vi "Execute.vi"(8 "error in (no error)":errorcluster, 10 "System In":refnum<class "abs_System.lvclass">, 11 "Node in":refnum<class "Test Double Float.lvclass">) -> (0 "error out":errorcluster, 1 "Status":T1, 2 "System Out":refnum<class "abs_System.lvclass">, 3 "Node out":refnum<class "Test Double Float.lvclass">)   [LabVIEW 2021, in "BT.lvlib" / "Test Double Float.lvclass"]
uses:
  Test Double Float.lvclass
  C:/Users/Tim/Documents/LabVIEW/2021/Behaviour Tree/Source/abs_Type Leaf/abs_Type Leaf.lvclass
  abs_Node/Status.ctl
  abs_System/abs_System.lvclass
  LV_Abstract/Source/Abs_Types/Double Float/Abs_Double Float.lvclass
  C:/Users/Tim/Documents/GitHub/LV_Abstract/Source/Abs_Types/Type/Abs_Type.lvclass
  abs_Type Leaf/abs_Type Leaf.lvclass/abs_Type Leaf.ctl
  Test Double Float.lvclass/Test Double Float.ctl
  abs_Type Leaf/Properties/Read Value Class.vi
  Properties/Read Lower Limit.vi
  Properties/Read Upper Limit.vi
  Properties/Read Limit Test Type.vi
  abs_Type Leaf/Properties/Write Value Class.vi
  LV_Abstract/Source/Abs_Types/Type/Abs_Type.lvclass
  abs_Type Leaf/abs_Type Leaf.lvclass
  abs_Node/abs_Node.lvclass
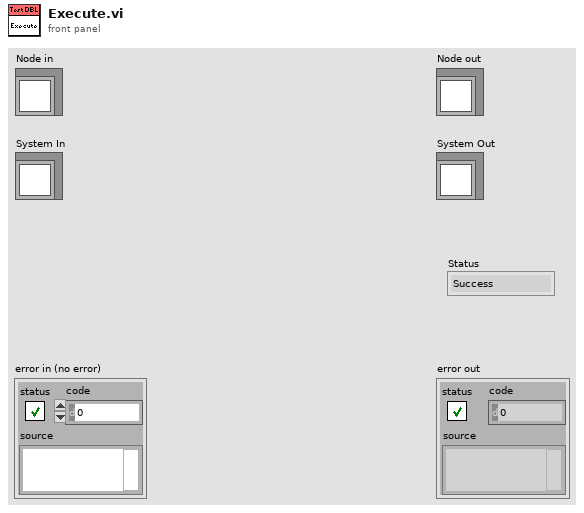
[diagram p1: front panel]
types:
  T1 = typedef "BT.lvlib/abs_Node.lvclass/Status.ctl" = enum16{"Success", "Failure", "Running"}
  T2 = typedef "BT.lvlib/Limit Test Type.ctl" = enum16{"x == Lo", "x != Lo", "x > Lo", "x < Lo", "x >= Lo", "x <= Lo", "Lo > x < Hi", "Lo >= x <= Hi", "Lo >= x < Hi", "Lo > x <= Hi", "Lo < x > Hi", "Lo <= x >= Hi", "Lo <= x > Hi", "Lo < x >= Hi", "x == Lo +/- Hi"}
  T3 = typedef "Abs_Double Float.lvclass/Type.ctl" = dbl
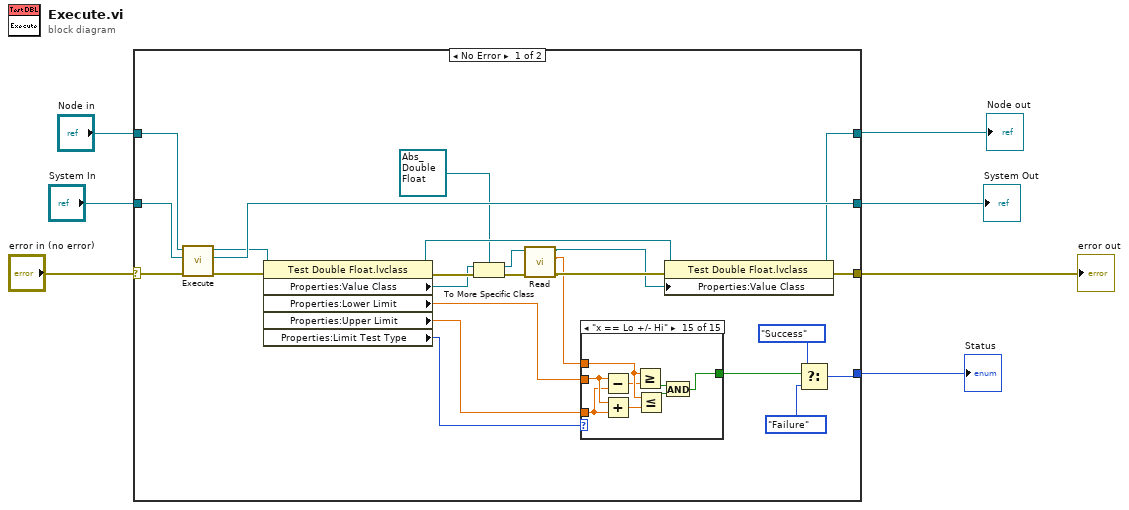
[diagram p0: block diagram]
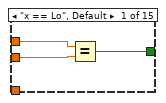
[diagram p2: hidden frame]
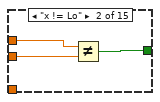
[diagram p3: hidden frame]
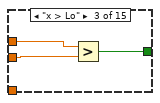
[diagram p4: hidden frame]
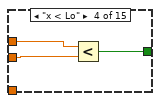
[diagram p5: hidden frame]
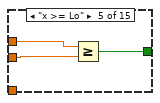
[diagram p6: hidden frame]
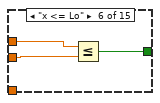
[diagram p7: hidden frame]
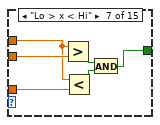
[diagram p8: hidden frame]
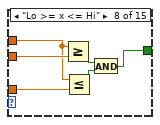
[diagram p9: hidden frame]
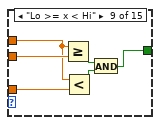
[diagram p10: hidden frame]
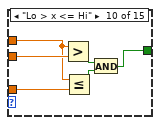
[diagram p11: hidden frame]
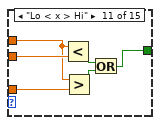
[diagram p12: hidden frame]
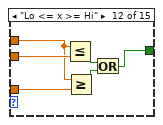
[diagram p13: hidden frame]
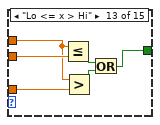
[diagram p14: hidden frame]
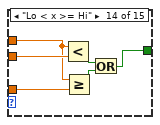
[diagram p15: hidden frame]
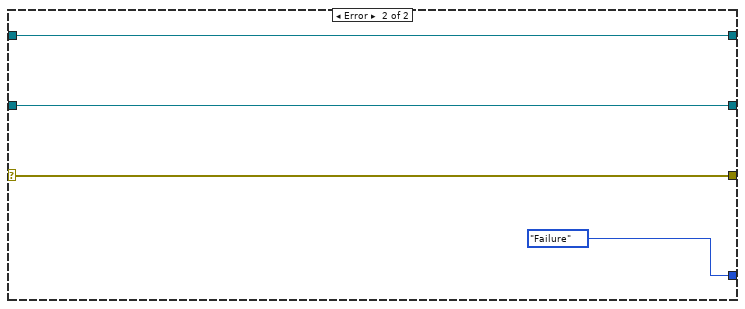
[diagram p16: hidden frame]
diagram:
  n1 = case shown="No Error" "error in (no error)" {
    selector: "error in (no error)" -> [w30 w107]
    tunnel: [w31 w108] -> w2
    tunnel: "System In" -> [w29 w108]
    tunnel: "Node in" -> [w28 w109]
    tunnel: [w24 w107] -> w4
    tunnel: [w23 w109] -> w1
    tunnel: [w20 Status."Failure" ("Status")] -> w3
    frame No Error {
      n2 = call-parent "Execute.vi"("error in (no error)"=w30, "System In"=w29, "Node in"=w28) -> ("error out"=w27:errorcluster, "System Out"=w31:refnum<class "abs_System.lvclass">, "Node out"=w26:refnum<class "Test Double Float.lvclass">)  [unwired: 5 in, 1 out]
      n3 = property class="Test Double Float.lvclass"(reference=w26, error in=w27) -> (reference out=w25:refnum<class "Test Double Float.lvclass">, error out=w11:errorcluster, "Properties:Value Class"=w10:refnum<class "Abs_Type.lvclass">, "Properties:Lower Limit"=w19:dbl, "Properties:Upper Limit"=w16:dbl, "Properties:Limit Test Type"=w17:T2)
      n4 = To More Specific Class(target class=refnum<class "Abs_Double Float.lvclass"> refnum ("Double Float.lvclass_340760 in"), reference=w10, error in=w11) -> (specific class reference=w8:refnum<class "Abs_Double Float.lvclass">, error out=w12:errorcluster)
      n5 = call-dynamic "Read.vi"("error in (no error)"=w12, "Double Float.lvclass_340760 in"=w8) -> ("error out"=w15:errorcluster, "Value"=w14:T3, "Double Float.lvclass_340760 out"=w13:refnum<class "Abs_Double Float.lvclass">)  [unwired: 7 in]
      n6 = case shown="\"x == Lo +/- Hi\"" w17 {
        tunnel: w14 -> [w33 w37 w40 w43 w46 w49 w54 w60 w66 w72 w78 w84 w90 w96 w105]
        tunnel: w19 -> [w34 w36 w39 w42 w45 w48 w55 w61 w67 w73 w79 w85 w91 w97 w100]
        tunnel: [w32 w35 w38 w41 w44 w47 w50 w56 w62 w68 w74 w80 w86 w92 w102] -> w18
        tunnel: w16 -> [_ _ _ _ _ _ w53 w59 w65 w71 w77 w83 w89 w95 w99]
        frame "x == Lo", Default {
          n7 = Equal?(x=w33, y=w34) -> (x = y?=w32:bool)
        }
        frame "x != Lo" {
          n8 = Not Equal?(x=w37, y=w36) -> (x != y?=w35:bool)
        }
        frame "x > Lo" {
          n9 = Greater?(x=w40, y=w39) -> (0:w38:bool)
        }
        frame "x < Lo" {
          n10 = Less?(x=w43, y=w42) -> (x < y?=w41:bool)
        }
        frame "x >= Lo" {
          n11 = Greater Or Equal?(x=w46, y=w45) -> (x >= y?=w44:bool)
        }
        frame "x <= Lo" {
          n12 = Less Or Equal?(x=w49, y=w48) -> (x <= y?=w47:bool)
        }
        frame "Lo > x < Hi" {
          n13 = Greater?(x=w54, y=w55) -> (0:w52:bool)
          n14 = Less?(x=w54, y=w53) -> (x < y?=w51:bool)
          n15 = And(x=w52, y=w51) -> (x .and. y?=w50:bool)
        }
        frame "Lo >= x <= Hi" {
          n16 = Greater Or Equal?(x=w60, y=w61) -> (x >= y?=w58:bool)
          n17 = Less Or Equal?(x=w60, y=w59) -> (x <= y?=w57:bool)
          n18 = And(x=w58, y=w57) -> (x .and. y?=w56:bool)
        }
        frame "Lo >= x < Hi" {
          n19 = Greater Or Equal?(x=w66, y=w67) -> (x >= y?=w64:bool)
          n20 = Less?(x=w66, y=w65) -> (x < y?=w63:bool)
          n21 = And(x=w64, y=w63) -> (x .and. y?=w62:bool)
        }
        frame "Lo > x <= Hi" {
          n22 = Greater?(x=w72, y=w73) -> (0:w70:bool)
          n23 = Less Or Equal?(x=w72, y=w71) -> (x <= y?=w69:bool)
          n24 = And(x=w70, y=w69) -> (x .and. y?=w68:bool)
        }
        frame "Lo < x > Hi" {
          n25 = Less?(x=w78, y=w79) -> (x < y?=w76:bool)
          n26 = Greater?(x=w78, y=w77) -> (0:w75:bool)
          n27 = Or(x=w76, y=w75) -> (x .or. y?=w74:bool)
        }
        frame "Lo <= x >= Hi" {
          n28 = Less Or Equal?(x=w84, y=w85) -> (x <= y?=w82:bool)
          n29 = Greater Or Equal?(x=w84, y=w83) -> (x >= y?=w81:bool)
          n30 = Or(x=w82, y=w81) -> (x .or. y?=w80:bool)
        }
        frame "Lo <= x > Hi" {
          n31 = Less Or Equal?(x=w90, y=w91) -> (x <= y?=w88:bool)
          n32 = Greater?(x=w90, y=w89) -> (0:w87:bool)
          n33 = Or(x=w88, y=w87) -> (x .or. y?=w86:bool)
        }
        frame "Lo < x >= Hi" {
          n34 = Less?(x=w96, y=w97) -> (x < y?=w94:bool)
          n35 = Greater Or Equal?(x=w96, y=w95) -> (x >= y?=w93:bool)
          n36 = Or(x=w94, y=w93) -> (x .or. y?=w92:bool)
        }
        frame "x == Lo +/- Hi" {
          n37 = Subtract(x=w100, y=w99) -> (x-y=w101:dbl)
          n38 = Add(x=w100, y=w99) -> (x+y=w98:dbl)
          n39 = Greater Or Equal?(x=w105, y=w101) -> (x >= y?=w104:bool)
          n40 = Less Or Equal?(x=w105, y=w98) -> (x <= y?=w103:bool)
          n41 = And(x=w104, y=w103) -> (x .and. y?=w102:bool)
        }
      }
      n42 = property class="Test Double Float.lvclass"(reference=w25, error in=w15, "Properties:Value Class"=w13) -> (reference out=w23:refnum<class "Test Double Float.lvclass">, error out=w24:errorcluster)
      n43 = Select(t=Status."Success" ("Status"), s=w18, f=Status."Failure") -> (s? t:f=w20:T1)
    }
    frame Error {
    }
  }
  "error out" <- w4
  "Node out" <- w1
  "Status" <- w3
  "System Out" <- w2
